vi "ColorAPI_GetData.vi"(8 "错误输入（无错误）":errorcluster) -> (0 "错误输出":errorcluster, 1 "Blue":i32, 2 "Green":i32, 3 "Red":i32)   [LabVIEW 2011, in "ColorSensorlib.lvlib"]
uses:
  ColorSensorlib.lvlib
  ColorDis.dll
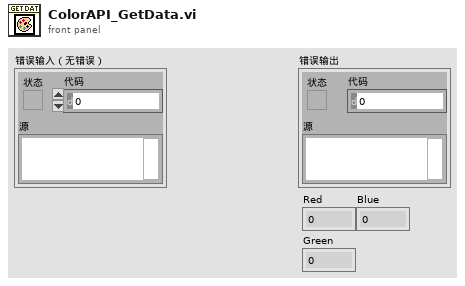
[diagram p1: front panel]
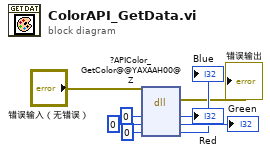
[diagram p0: block diagram]
diagram:
  n1 = dll-call lib="PTH1Cabs D\tDocumentsDesktop颜色传感器LabViewColorDis.dll" fn="?APIColor_GetColor@@YAXAAH00@Z"(error in="错误输入（无错误）", "Red"=0, "Green"=0, "Blue"=0) -> (error out=→"错误输出":errorcluster, "Red"=→"Red":i32, "Green"=→"Green":i32, "Blue"=→"Blue":i32)  [unwired: 3 in, 1 out]
